vi "Relay_Button.vi"() -> ()   [LabVIEW 2022 SP3]
uses:
  <vilib>/Instr/_visa.llb/VISA Configure Serial Port (Instr).vi
panel:
  in  "Left":bool
  in  "Down":bool
  in  "Up":bool
  in  "Right":bool
  in  "Adjustor Number":dbl
  in  "Relay On/Off":bool
  in  "Emergency Stop":bool
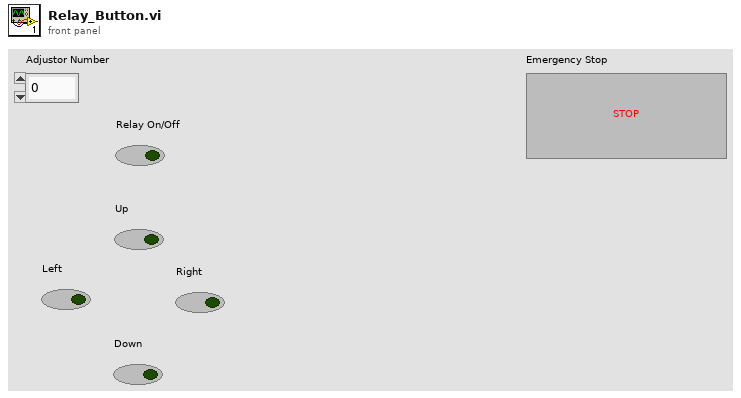
[diagram p1: front panel]
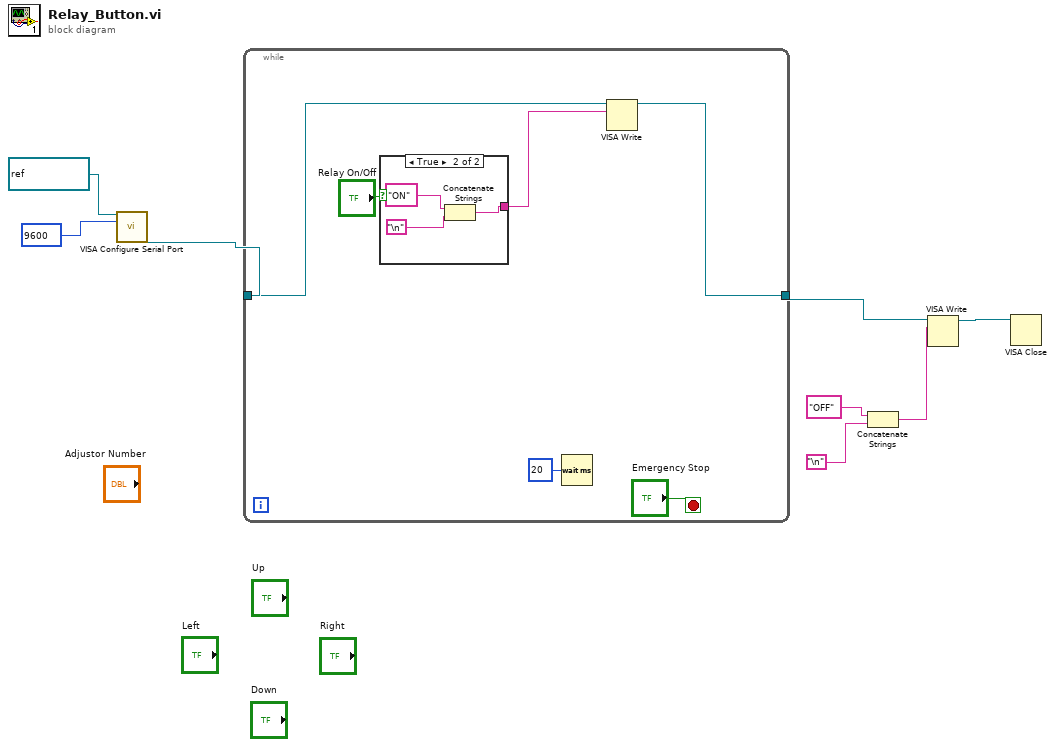
[diagram p0: block diagram]
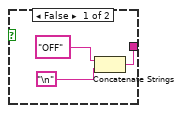
[diagram p2: hidden frame]
diagram:
  n1 = call-poly "VISA Configure Serial Port"("VISA resource name"=refnum<visa-resource-name> "COM8", "baud rate (9600)"=u32 9600) -> ("VISA resource name out"=w1:refnum<visa-resource-name>)  [unwired: 12 in, 1 out]
  n2 = while {
    tunnel: w1 -> [w9]
    tunnel: [w12] -> w6
    stop <- "Emergency Stop" stop-if-true
    n3 = case shown="True" "Relay On/Off" {
      tunnel: [w15 w18] -> w10
      frame False {
        n4 = Concatenate Strings("OFF", "\n") -> (w15:string)
      }
      frame True {
        n5 = Concatenate Strings("ON", "\n") -> (w18:string)
      }
    }
    n6 = Wait (ms)(milliseconds to wait=u32 20) -> ()  [unwired: 1 out]
    n7 = VISA Write(VISA resource name=w9, write buffer=w10) -> (VISA resource name out=w12:refnum<visa-resource-name>)  [unwired: 1 in, 2 out]
  }
  n8 = Concatenate Strings("OFF", "\n") -> (w2:string)
  n9 = VISA Write(VISA resource name=w6, write buffer=w2) -> (VISA resource name out=w5:refnum<visa-resource-name>)  [unwired: 1 in, 2 out]
  n10 = VISA Close(VISA resource name=w5) -> ()  [unwired: 1 in, 1 out]
